vi "Large Signal Bench control panel.vi"() -> ()   [LabVIEW 2020]
uses:
  <vilib>/DAQmx/read.llb/DAQmx Read (Digital Bool 1Line 1Point).vi
  <vilib>/DAQmx/write.llb/DAQmx Write (Digital Bool 1Line 1Point).vi
  <vilib>/DAQmx/miscellaneous.llb/DAQmx Fill In Error Info.vi
  Instruments/Path Switch/NI USB-6501/NI USB-6501.lvclass
panel:
  in  "System Refresh Button":bool
  in  "System Stop Button":bool
  out "PA2-temp sensor":bool
  in  "SG1 switch ctrl1":bool
  in  "SG1 switch ctrl0":bool
  in  "SG1 switch Vdd":bool
  in  "PA2 power":bool
  in  "DUT4SWITCH":bool caption="DUT-selector.RF4"
  in  "DUT3SWITCH":bool caption="DUT-selector.RF3"
  in  "DUT2SWITCH":bool caption="DUT-selector.RF2"
  in  "SA PATH SELECTOR":enum32{"IMD", "Harmonics"}(radio) caption="Spectrum Analyzer path selector"
  in  "DUT1SWITCH":bool caption="DUT-selector.RF1"
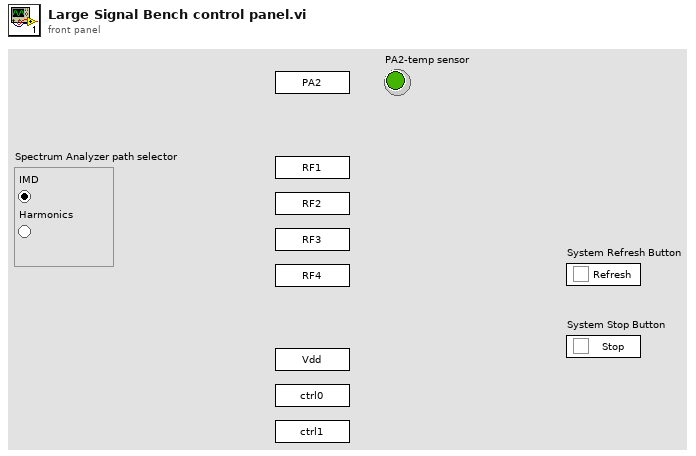
[diagram p1: front panel]
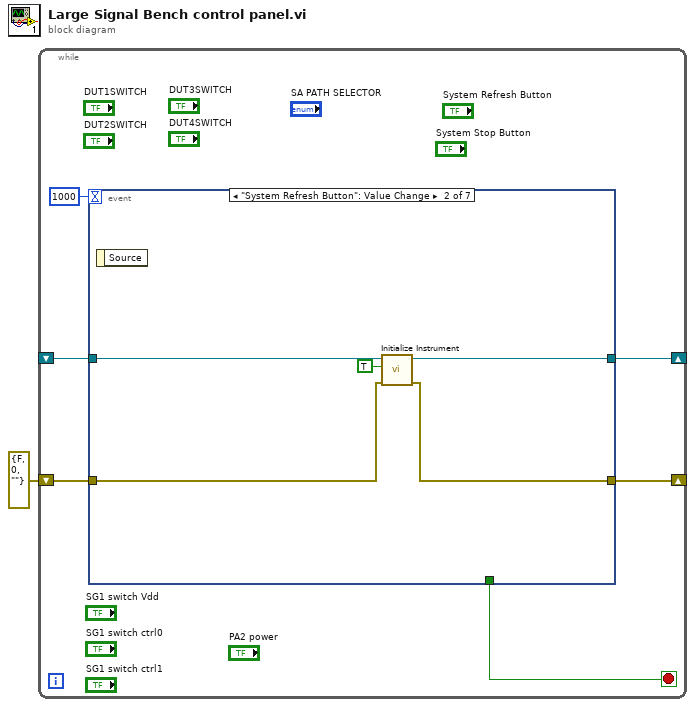
[diagram p0: block diagram]
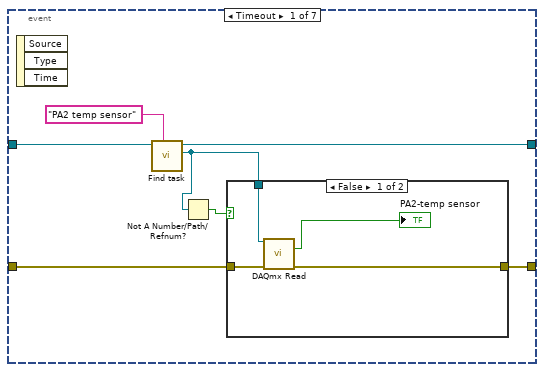
[diagram p2: hidden frame]
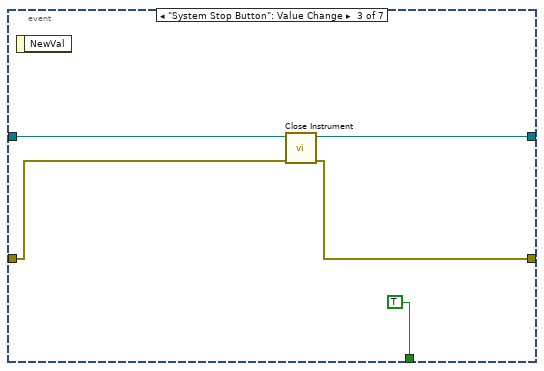
[diagram p4: hidden frame]
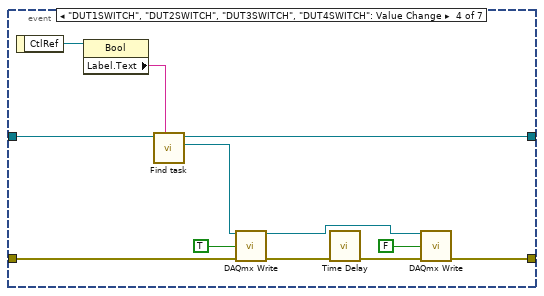
[diagram p5: hidden frame]
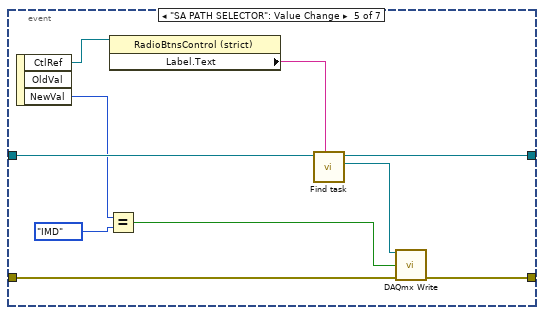
[diagram p6: hidden frame]
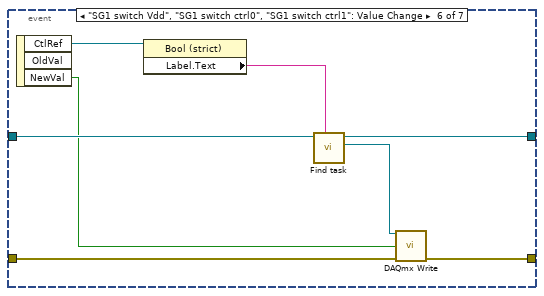
[diagram p7: hidden frame]
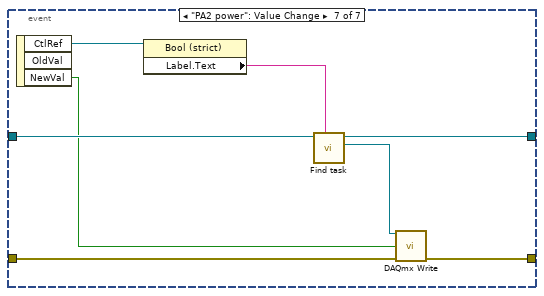
[diagram p8: hidden frame]
diagram:
  n1 = while {
    shift-right: [w5] -> _
    shift-left: _ -> [w7]
    shift-right: [w3] -> _
    shift-left: errorcluster {"status"=FALSE, "code"=0, "source"=""} ("error out") -> [w2]
    stop <- w6 stop-if-true
    n2 = event shown="[1] \"System Refresh Button\": Value Change" {
      selector: _ -> [_ _ _ _ _ _ _]
      dyn-events: _ -> [_ _ _ _ _ _ _]
      timeout: 1000 -> [_ _ _ _ _ _ _]
      tunnel: w7 -> [w14 w23 w28 w39 w49 w57 w65]
      tunnel: [w13 w24 w27 w38 w48 w56 w64] -> w5
      tunnel: [_ _ TRUE _ _ _ _] -> w6
      tunnel: [w11 w22 w25 w35 w47 w55 w63] -> w3
      tunnel: w2 -> [w10 w21 w26 w34 w46 w54 w62]
      event Timeout {
        n3 = event-data() -> ()  [unwired: 1 in, 3 out]
        n4 = call "Find task.vi"("Function"="PA2 temp sensor", "NI USB-6501 in"=w14) -> ("Task"=w9:refnum<k21>, "NI USB-6501 out"=w13:refnum<class "NI USB-6501.lvclass">)  [unwired: 7 in, 1 out]
        n5 = Not A Number/Path/Refnum?(number/path/refnum=w9) -> (NaN/Path/Refnum?=w8:bool)
        n6 = case shown="False" w8 {
          tunnel: w9 -> [w18 _]
          tunnel: [w17 w19] -> w11
          tunnel: w10 -> [w16 w19]
          frame False {
            n7 = call-poly <vilib>:"DAQmx Read.vi"("task/channels in"=w18, "error in"=w16) -> ("data"=→"PA2-temp sensor":bool, "error out"=w17:errorcluster)  [unwired: 11 in, 1 out]
          }
          frame True {
          }
        }
      }
      event "System Refresh Button": Value Change {
        n8 = event-data() -> ()  [unwired: 1 in, 1 out]
        n9 = call-dynamic "Initialize Instrument.vi"("error in (no error)"=w21, "Reset"=TRUE, "NI USB-6501 in"=w23) -> ("error out"=w22:errorcluster, "NI USB-6501 out"=w24:refnum<class "NI USB-6501.lvclass">)  [unwired: 7 in]
      }
      event "System Stop Button": Value Change {
        n10 = event-data() -> ()  [unwired: 1 in, 1 out]
        n11 = call-dynamic "Close Instrument.vi"("error in (no error)"=w26, "NI USB-6501 in"=w28) -> ("error out"=w25:errorcluster, "NI USB-6501 out"=w27:refnum<class "NI USB-6501.lvclass">)  [unwired: 8 in]
      }
      event "DUT1SWITCH", "DUT2SWITCH", "DUT3SWITCH", "DUT4SWITCH": Value Change {
        n12 = event-data() -> ("CtlRef"=w41:refnum<vi>)  [unwired: 1 in]
        n13 = property class="Bool"(reference=w41) -> ("Label.Text"=w40:string)  [unwired: 1 in, 2 out]
        n14 = call "Find task.vi"("Function"=w40, "NI USB-6501 in"=w39) -> ("Task"=w33:refnum<k21>, "NI USB-6501 out"=w38:refnum<class "NI USB-6501.lvclass">)  [unwired: 7 in, 1 out]
        n15 = call-poly <vilib>:"DAQmx Write.vi"("task/channels in"=w33, "data"=TRUE, "error in"=w34) -> ("task out"=w32:refnum<k21>, "error out"=w37:errorcluster)  [unwired: 10 in, 1 out]
        n16 = call "Time Delay"("error in (no error)"=w37) -> ("error out"=w36:errorcluster)  [unwired: 10 in]
        n17 = call-poly <vilib>:"DAQmx Write.vi"("task/channels in"=w32, "data"=FALSE, "error in"=w36) -> ("error out"=w35:errorcluster)  [unwired: 10 in, 2 out]
      }
      event "SA PATH SELECTOR": Value Change {
        n18 = event-data() -> ("CtlRef"=w51:refnum<vi>, "NewVal"=w43:enum32{"IMD", "Harmonics"})  [unwired: 1 in, 1 out]
        n19 = Equal?(x=w43, y=enum32{"IMD", "Harmonics"}."IMD" ("SA PATH SELECTOR")) -> (x = y?=w42:bool)
        n20 = property class="RadioBtnsControl (strict)"(reference=w51) -> ("Label.Text"=w50:string)  [unwired: 1 in, 2 out]
        n21 = call "Find task.vi"("Function"=w50, "NI USB-6501 in"=w49) -> ("Task"=w45:refnum<k21>, "NI USB-6501 out"=w48:refnum<class "NI USB-6501.lvclass">)  [unwired: 7 in, 1 out]
        n22 = call-poly <vilib>:"DAQmx Write.vi"("task/channels in"=w45, "data"=w42, "error in"=w46) -> ("error out"=w47:errorcluster)  [unwired: 10 in, 2 out]
      }
      event "SG1 switch Vdd", "SG1 switch ctrl0", "SG1 switch ctrl1": Value Change {
        n23 = event-data() -> ("CtlRef"=w59:refnum<vi>, "NewVal"=w52:bool)  [unwired: 1 in, 1 out]
        n24 = property class="Bool (strict)"(reference=w59) -> ("Label.Text"=w58:string)  [unwired: 1 in, 2 out]
        n25 = call "Find task.vi"("Function"=w58, "NI USB-6501 in"=w57) -> ("Task"=w53:refnum<k21>, "NI USB-6501 out"=w56:refnum<class "NI USB-6501.lvclass">)  [unwired: 7 in, 1 out]
        n26 = call-poly <vilib>:"DAQmx Write.vi"("task/channels in"=w53, "data"=w52, "error in"=w54) -> ("error out"=w55:errorcluster)  [unwired: 10 in, 2 out]
      }
      event "PA2 power": Value Change {
        n27 = event-data() -> ("CtlRef"=w67:refnum<vi>, "NewVal"=w60:bool)  [unwired: 1 in, 1 out]
        n28 = property class="Bool (strict)"(reference=w67) -> ("Label.Text"=w66:string)  [unwired: 1 in, 2 out]
        n29 = call "Find task.vi"("Function"=w66, "NI USB-6501 in"=w65) -> ("Task"=w61:refnum<k21>, "NI USB-6501 out"=w64:refnum<class "NI USB-6501.lvclass">)  [unwired: 7 in, 1 out]
        n30 = call-poly <vilib>:"DAQmx Write.vi"("task/channels in"=w61, "data"=w60, "error in"=w62) -> ("error out"=w63:errorcluster)  [unwired: 10 in, 2 out]
      }
    }
  }
